vi "Write configured channels.vi"(8 "error in":errorcluster, 10 "configured channels":refnum<class "TBM channel.lvclass">[](array[class]), 11 "fixed channel tag bus module configuration in":refnum<class "fixed channel tag bus module configuration.lvclass">) -> (0 "error out":errorcluster, 3 "fixed channel tag bus module configuration out":refnum<class "fixed channel tag bus module configuration.lvclass">)   [LabVIEW 2013, in "fixed channel tag bus module configuration.lvclass"]
uses:
  fixed channel tag bus module configuration.lvclass
  <vilib>/NI/Tag Bus Module Framework/channel/TBM channel.lvclass
  fixed channel tag bus module configuration.lvclass/fixed channel tag bus module configuration.ctl
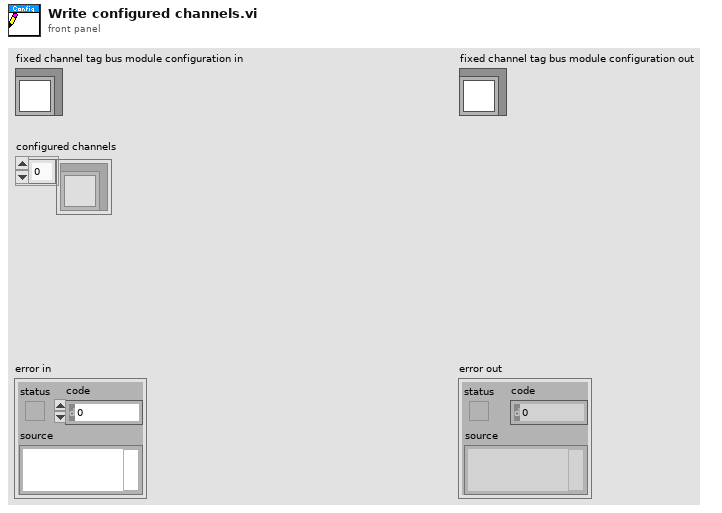
[diagram p1: front panel]
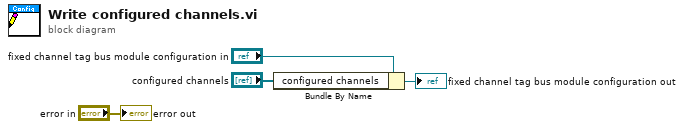
[diagram p0: block diagram]
diagram:
  n1 = Bundle By Name(cluster="fixed channel tag bus module configuration in", "configured channels"="configured channels") -> (→"fixed channel tag bus module configuration out":refnum<class "fixed channel tag bus module configuration.lvclass">)
  "error out" <- "error in"
